vi "SwissSPAD Live_Compute SS3 Gate Characteristics.vi"(7 "Gate Characteristics Refnum":refnum<vi>, 8 "Error In":errorcluster, 11 "SS3 DAQ Parameters":T2={"10 bits"=FALSE, "# Exposure Sequences"=0, "# 1-bit Frame per Gate"=255, "Gate Shift"=0, "# Gate Pairs per Set"=0, "# Sets"=1, "Laser Period"=0.0, "Sync Period"=0.0, "Gate Offset"=0, "Auto-adjust Gate Offset"=FALSE, "Gate Definition"={"gs_psincdec_0"=0, "gs_psincdec_1"=0, "gs_no_shift_adj_1"=0, "gate_adj_2"=0}, "Gate Width (ns)"=0.0, "Reversed Shift"=FALSE, "Intensity Mode"=FALSE, "Gate Definition Mode"=enum."Item 0"} {"Gate Width (ns)" min=0.0 max=100.0 format="%#_5g"; "# Sets" min=1}) -> (0 "Error Out":errorcluster, 3 "Gate Characteristics":T1)   [LabVIEW 2021]
uses:
  SwissSPAD Live_SS3 DAQ Parameters.ctl
  SwissSPAD Live_SS3 Gate Definition.ctl
  SS3 Gate Width Definition Mode.ctl
  SwissSPAD Live_Gate Characteristics.ctl
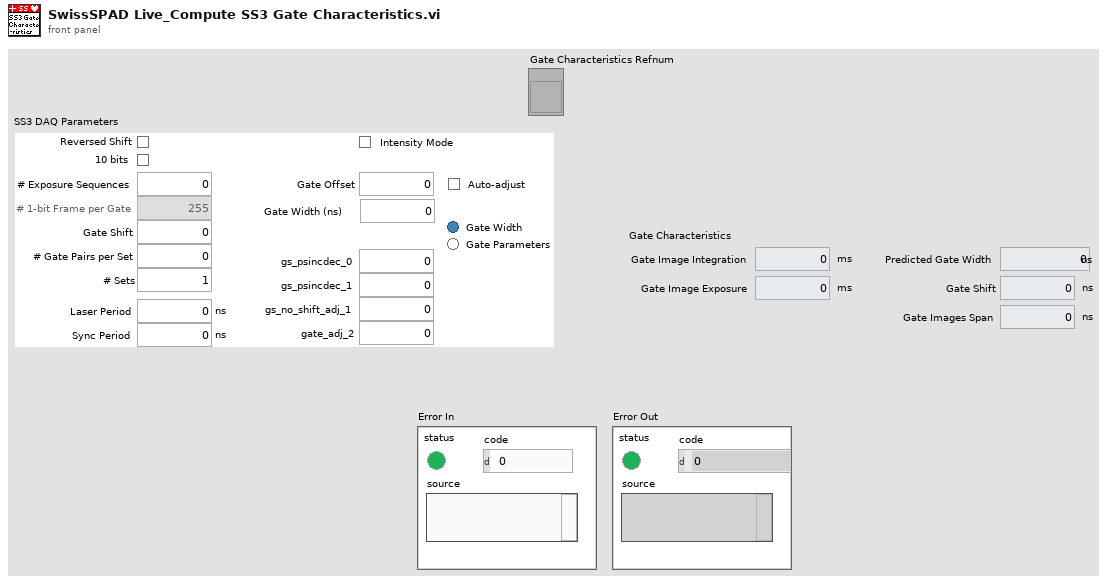
[diagram p1: front panel]
types:
  T1 = typedef "SwissSPAD Live_Gate Characteristics.ctl" = cluster{"Predicted Gate Width":dbl[unit], "Gate Image Integration":dbl[unit], "Gate Image Exposure":dbl[unit], "Gate Shift":dbl[unit], "Gate Images Span":dbl[unit]}
  T2 = typedef "SwissSPAD Live_SS3 DAQ Parameters.ctl" = cluster{"10 bits":bool, "# Exposure Sequences":u32, "# 1-bit Frame per Gate":u32, "Gate Shift":u32, "# Gate Pairs per Set":u32, "# Sets":u32, "Laser Period":dbl[unit], "Sync Period":dbl[unit], "Gate Offset":u32, "Auto-adjust Gate Offset":bool, "Gate Definition":T3, "Gate Width (ns)":dbl, "Reversed Shift":bool, "Intensity Mode":bool, "Gate Definition Mode":T4}
  T3 = typedef "SwissSPAD Live_SS3 Gate Definition.ctl" = cluster{"gs_psincdec_0":u32, "gs_psincdec_1":u32, "gs_no_shift_adj_1":u32, "gate_adj_2":u32}
  T4 = typedef "SS3 Gate Width Definition Mode.ctl" = enum32{"Item 0", "Item 1"}
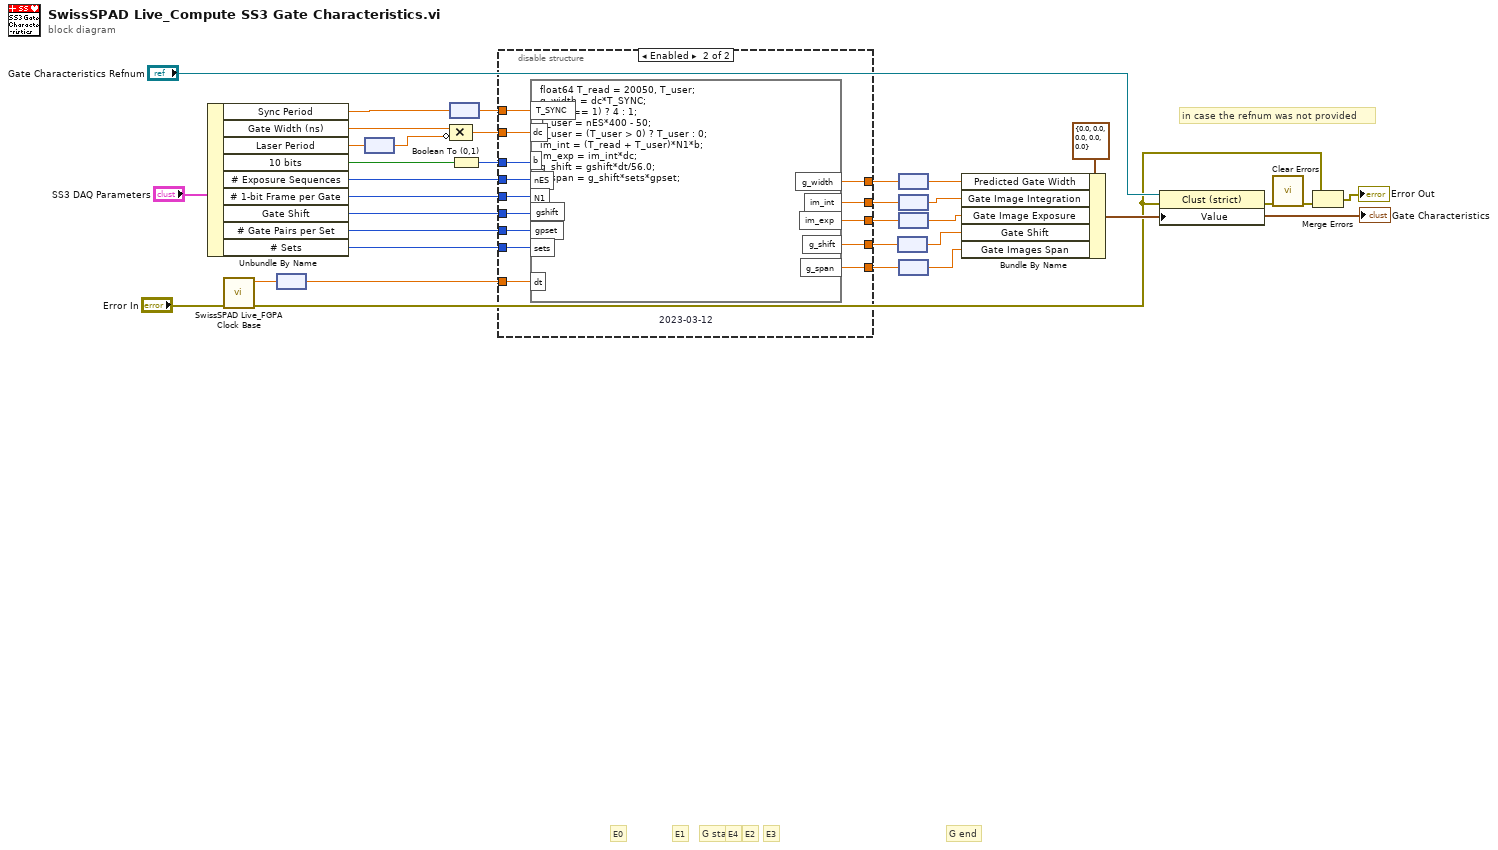
[diagram p0: block diagram]
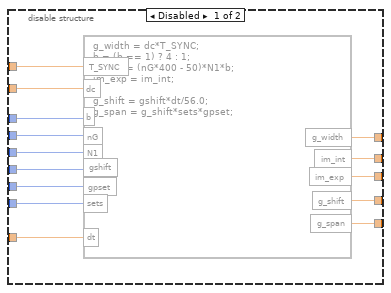
[diagram p2: hidden frame]
diagram:
  # "in case the refnum was not provided"
  # "G end"
  # "G start"
  # "E0"
  # "E4"
  # "E3"
  # "E2"
  # "E1"
  n1 = Unbundle By Name("SS3 DAQ Parameters") -> ("Sync Period"=w9:dbl[unit], "Gate Width (ns)"=w34:dbl, "Laser Period"=w2:dbl[unit], "10 bits"=w31:bool, "# Exposure Sequences"=w29:u32, "# 1-bit Frame per Gate"=w28:u32, "Gate Shift"=w21:u32, "# Gate Pairs per Set"=w16:u32, "# Sets"=w15:u32)
  n2 = call "SwissSPAD Live_FGPA Clock Base.vi"("error in (no error)"="Error In") -> ("error out"=w6:errorcluster, "Clock Base"=w5:dbl[unit])  [unwired: 9 in]
  n3 = node(w5) -> (w4:dbl)
  n4 = node(w2) -> (w1:dbl)
  n5 = node(w9) -> (w8:dbl)
  n6 = Compound Arithmetic op=MULTIPLY(w34, invert w1) -> (w3:dbl)
  n7 = Boolean To (0,1)(Boolean=w31) -> (0, 1=w30:i16)
  n8 = disable-structure shown="Enabled" {
    disable-tunnel: [w48 w62] -> w33
    disable-tunnel: w30 -> [w47 w61]
    disable-tunnel: w29 -> [w46 w60]
    disable-tunnel: w28 -> [w45 w59]
    disable-tunnel: [w44 w58] -> w27
    disable-tunnel: [w43 w57] -> w26
    disable-tunnel: w21 -> [w42 w56]
    disable-tunnel: [w41 w55] -> w20
    disable-tunnel: [w40 w54] -> w18
    disable-tunnel: w16 -> [w39 w53]
    disable-tunnel: w15 -> [w38 w52]
    disable-tunnel: w8 -> [w37 w51]
    disable-tunnel: w4 -> [w36 w50]
    disable-tunnel: w3 -> [w35 w49]
    frame Disabled {
      n9 = formula code="g_width = dc*T_SYNC;\nb = (b == 1) ? 4 : 1;\nim_int = (nG*400 - 50)*N1*b;\nim_exp = im_int;\n\ng_shift = gshift*dt/56.0;\ng_span = g_shift*sets*gpset;"("dc"=w35, "b"=w47, "nG"=w46, "N1"=w45, "gshift"=w42, "gpset"=w39, "sets"=w38, "T_SYNC"=w37, "dt"=w36) -> ("g_width"=w48:dbl, "im_int"=w44:dbl, "im_exp"=w43:dbl, "g_shift"=w41:dbl, "g_span"=w40:dbl)
    }
    frame Enabled {
      n10 = formula code="float64 T_read = 20050, T_user;\ng_width = dc*T_SYNC;\nb = (b == 1) ? 4 : 1;\nT_user = nES*400 - 50;\nT_user = (T_user > 0) ? T_user : 0;\nim_int = (T_read + T_user)*N1*b;\nim_exp = im_int*dc;\ng_shift = gshift*dt/56.0;\ng_span = g_shift*sets*gpset;" "2023-03-12"("dc"=w49, "b"=w61, "nES"=w60, "N1"=w59, "gshift"=w56, "gpset"=w53, "sets"=w52, "T_SYNC"=w51, "dt"=w50) -> ("g_width"=w62:dbl, "im_int"=w58:dbl, "im_exp"=w57:dbl, "g_shift"=w55:dbl, "g_span"=w54:dbl)
    }
  }
  n11 = node(w20) -> (w19:dbl[unit])
  n12 = node(w33) -> (w24:dbl[unit])
  n13 = node(w27) -> (w23:dbl[unit])
  n14 = node(w26) -> (w22:dbl[unit])
  n15 = node(w18) -> (w17:dbl[unit])
  n16 = Bundle By Name(cluster=T1 {"Predicted Gate Width"=0.0, "Gate Image Integration"=0.0, "Gate Image Exposure"=0.0, "Gate Shift"=0.0, "Gate Images Span"=0.0} ("Gate Characteristics"), "Predicted Gate Width"=w24, "Gate Image Integration"=w23, "Gate Image Exposure"=w22, "Gate Shift"=w19, "Gate Images Span"=w17) -> (w12:T1)
  "Gate Characteristics" <- w12
  n17 = property class="Clust (strict)"(reference="Gate Characteristics Refnum", error in=w6, "Value"=w12) -> (error out=w13:errorcluster)  [unwired: 1 out]
  n18 = call <vilib>:"Clear Errors.vi"("error in (no error)"=w13) -> ("error out"=w11:errorcluster)  [unwired: 5 in, 1 out]
  n19 = Merge Errors(w6, w11) -> (→"Error Out":errorcluster)
